vi "MainControlLogic.vi"() -> ()   [LabVIEW 2014, in "UILib.lvlib"]
uses:
  UILib.lvlib
  <vilib>/Rock Robotics/WPI/Solenoid/WPI_SolenoidValue.ctl
  LiftLib/LiftLib.lvlib
  LatchLib/LatchLib.lvlib
  IntakeLib/IntakeLib.lvlib
  GateLib/GateLib.lvlib
panel:
  in  "Axes":dbl[](array[numeric])
  in  "POVs":i16[](array[numeric])
  in  "Buttons":bool[](array[boolean])
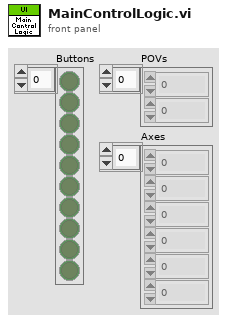
[diagram p1: front panel]
types:
  T1 = cluster{"Buttons[0]":bool, "Buttons[1]":bool, "Buttons[2]":bool, "Buttons[3]":bool, "Buttons[4]":bool, "Buttons[5]":bool, "Buttons[6]":bool, "Buttons[7]":bool, "Buttons[8]":bool}
  T2 = typedef "WPI_SolenoidValue.ctl" = enum16{"Off", "On", "Forward", "Reverse"}
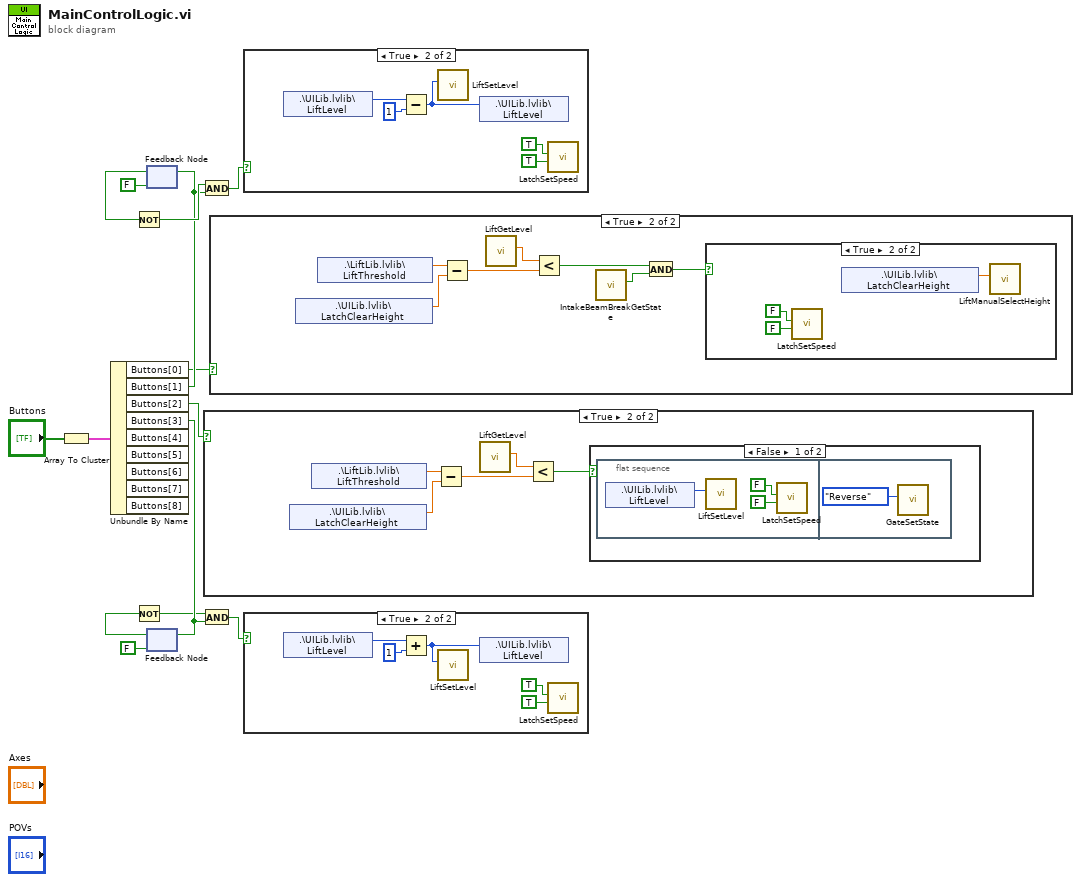
[diagram p0: block diagram]
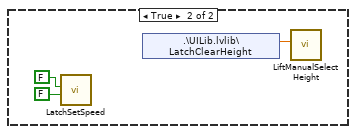
[diagram p3: hidden frame]
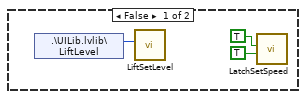
[diagram p5: hidden frame]
diagram:
  n1 = Array To Cluster(array="Buttons") -> (cluster=w13:T1)
  n2 = Unbundle By Name(w13) -> ("Buttons[0]"=w2:bool, "Buttons[1]"=w3:bool, "Buttons[2]"=w1:bool, "Buttons[3]"=w11:bool)  [unwired: 5 out]
  n3 = feedback #1(FALSE ("Buttons[3]")) -> (w6:bool)
  n4 = Not(x=w6) -> (.not. x?=w5:bool)
  n5 = feedback-in #1(w3) -> ()
  n6 = feedback-in #2(w11) -> ()
  n7 = feedback #2(FALSE ("Buttons[3]")) -> (w10:bool)
  n8 = Not(x=w10) -> (.not. x?=w9:bool)
  n9 = And(x=w5, y=w3) -> (x .and. y?=w4:bool)
  n10 = And(x=w9, y=w11) -> (x .and. y?=w8:bool)
  n11 = case shown="True" w1 {
    frame False {
    }
    frame True {
      n12 = shared-variable ".\\UILib.lvlib\\LatchClearHeight"() -> (w16:dbl)  [unwired: 1 in, 1 out]
      n13 = shared-variable ".\\LiftLib.lvlib\\LiftThreshold"() -> (w17:dbl)  [unwired: 1 in, 1 out]
      n14 = Subtract(x=w17, y=w16) -> (x-y=w19:dbl)
      n15 = call "LiftGetLevel.vi"() -> ("LiftCurrentHeight"=w18:dbl)  [unwired: 11 in]
      n16 = Less?(x=w18, y=w19) -> (x < y?=w15:bool)
      n17 = case shown="False" w15 {
        frame False {
          n18 = flat-sequence {
            frame #0 {
              n19 = shared-variable ".\\UILib.lvlib\\LiftLevel"() -> (w22:i32)  [unwired: 1 in, 1 out]
              n20 = call "LiftSetLevel.vi"("Index"=w22) -> ()  [unwired: 11 in]
              n21 = call "LatchSetSpeed.vi"("LatchContainerState"=FALSE, "LatchLatchState"=FALSE) -> ()  [unwired: 10 in]
            }
            frame #1 {
              n22 = call "GateSetState.vi"("GateCylState"=WPI_SolenoidValue."Reverse") -> ()  [unwired: 11 in]
            }
          }
        }
        frame True {
          n23 = call "LatchSetSpeed.vi"("LatchContainerState"=FALSE, "LatchLatchState"=FALSE) -> ()  [unwired: 10 in]
          n24 = shared-variable ".\\UILib.lvlib\\LatchClearHeight"() -> (w26:dbl)  [unwired: 1 in, 1 out]
          n25 = call "LiftManualSelectHeight.vi"("Height"=w26) -> ()  [unwired: 11 in]
        }
      }
    }
  }
  n26 = case shown="True" w2 {
    frame False {
    }
    frame True {
      n27 = shared-variable ".\\UILib.lvlib\\LatchClearHeight"() -> (w33:dbl)  [unwired: 1 in, 1 out]
      n28 = shared-variable ".\\LiftLib.lvlib\\LiftThreshold"() -> (w32:dbl)  [unwired: 1 in, 1 out]
      n29 = Subtract(x=w32, y=w33) -> (x-y=w30:dbl)
      n30 = call "LiftGetLevel.vi"() -> ("LiftCurrentHeight"=w31:dbl)  [unwired: 11 in]
      n31 = Less?(x=w31, y=w30) -> (x < y?=w29:bool)
      n32 = call "IntakeBeamBreakGetState.vi"() -> ("Switch Pressed"=w28:bool)  [unwired: 11 in]
      n33 = And(x=w29, y=w28) -> (x .and. y?=w27:bool)
      n34 = case shown="True" w27 {
        frame False {
          n35 = shared-variable ".\\UILib.lvlib\\LiftLevel"() -> (w34:i32)  [unwired: 1 in, 1 out]
          n36 = call "LiftSetLevel.vi"("Index"=w34) -> ()  [unwired: 11 in]
          n37 = call "LatchSetSpeed.vi"("LatchContainerState"=TRUE, "LatchLatchState"=TRUE) -> ()  [unwired: 10 in]
        }
        frame True {
          n38 = call "LatchSetSpeed.vi"("LatchContainerState"=FALSE, "LatchLatchState"=FALSE) -> ()  [unwired: 10 in]
          n39 = shared-variable ".\\UILib.lvlib\\LatchClearHeight"() -> (w39:dbl)  [unwired: 1 in, 1 out]
          n40 = call "LiftManualSelectHeight.vi"("Height"=w39) -> ()  [unwired: 11 in]
        }
      }
    }
  }
  n41 = case shown="True" w4 {
    frame False {
    }
    frame True {
      n42 = shared-variable ".\\UILib.lvlib\\LiftLevel"() -> (w44:i32)  [unwired: 1 in, 1 out]
      n43 = Subtract(x=w44, y=1) -> (x-y=w43:i32)
      n44 = call "LiftSetLevel.vi"("Index"=w43) -> ()  [unwired: 11 in]
      n45 = shared-variable ".\\UILib.lvlib\\LiftLevel"(w43) -> ()  [unwired: 1 in, 1 out]
      n46 = call "LatchSetSpeed.vi"("LatchContainerState"=TRUE, "LatchLatchState"=TRUE) -> ()  [unwired: 10 in]
    }
  }
  n47 = case shown="True" w8 {
    frame False {
    }
    frame True {
      n48 = shared-variable ".\\UILib.lvlib\\LiftLevel"() -> (w49:i32)  [unwired: 1 in, 1 out]
      n49 = Add(x=w49, y=1) -> (x+y=w47:i32)
      n50 = call "LiftSetLevel.vi"("Index"=w47) -> ()  [unwired: 11 in]
      n51 = shared-variable ".\\UILib.lvlib\\LiftLevel"(w47) -> ()  [unwired: 1 in, 1 out]
      n52 = call "LatchSetSpeed.vi"("LatchContainerState"=TRUE, "LatchLatchState"=TRUE) -> ()  [unwired: 10 in]
    }
  }
